vi "init.vi"(0 "VISA Refnum in":refnum<visa-resource-name>) -> (4 "VISA out":refnum<visa-resource-name>, 6 "client handle out":T2, 8 "Internet OK":bool, 10 "Cluster of queues":T1, 15 "VISA error out":errorcluster)   [LabVIEW 2016]
uses:
  <vilib>/httpClient/ClientHandle.ctl
  <vilib>/Utility/error.llb/DialogType.ctl
  <vilib>/Instr/_visa.llb/VISA Configure Serial Port (Instr).vi
  <vilib>/httpClient/LabVIEWHTTPClient.lvlib
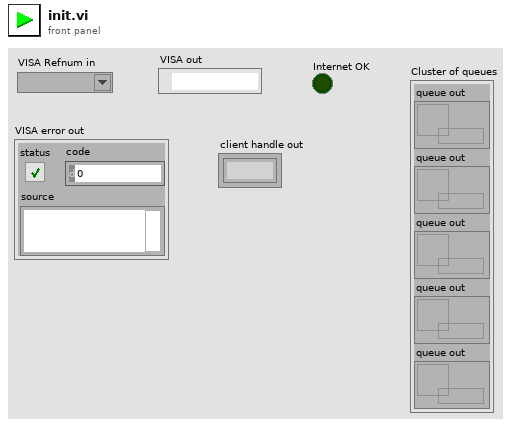
[diagram p1: front panel]
types:
  T1 = cluster{"queue out":refnum<queue>, "queue out":refnum<queue>, "queue out":refnum<queue>, "queue out":refnum<queue>, "queue out":refnum<queue>}
  T2 = typedef "LabVIEWHTTPClient.lvlib/ClientHandle.ctl" = refnum<k1>
  T3 = typedef "DialogType.ctl" = u16
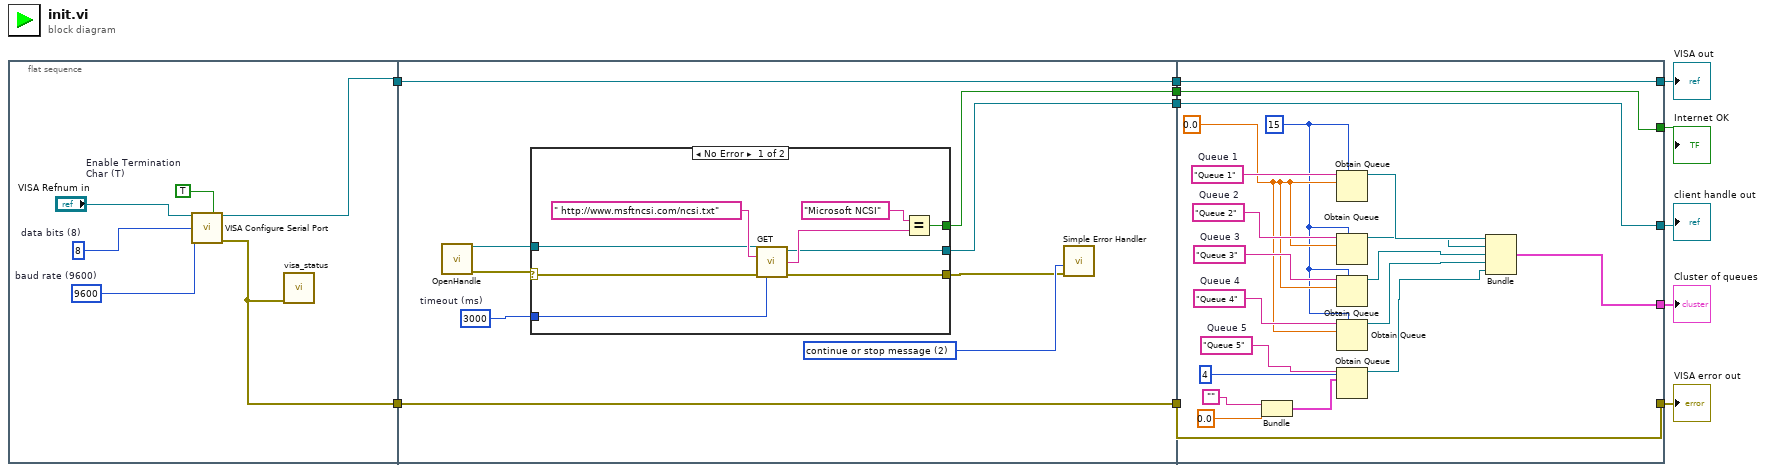
[diagram p0: block diagram]
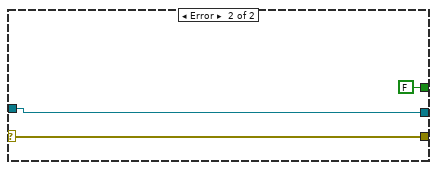
[diagram p2: hidden frame]
diagram:
  n1 = flat-sequence {
    tunnel: [w13] -> w11
    tunnel: [w12] -> w7
    tunnel: w11 -> [w21]
    tunnel: [w21] -> w10
    tunnel: [w20] -> w8
    tunnel: w7 -> [w20]
    tunnel: [w19] -> w5
    tunnel: [w18] -> w3
    tunnel: [w55] -> w9
    tunnel: w10 -> [w55]
    tunnel: [w54] -> w6
    tunnel: w8 -> [w54]
    tunnel: [w53] -> w4
    tunnel: w5 -> [w53]
    tunnel: [w52] -> w2
    tunnel: w3 -> [w52]
    tunnel: [w40] -> w1
    frame #0 {
      w14 = u16 8  # data bits (8)
      w15 = TRUE  # Enable Termination Char (T)
      w16 = u32 9600  # baud rate (9600)
      n2 = call-poly "VISA Configure Serial Port"("VISA resource name"="VISA Refnum in", "Enable Termination\nChar (T)"=w15, "baud rate (9600)"=w16, "data bits (8)"=w14) -> ("VISA resource name out"=w13:refnum<visa-resource-name>, "error out"=w12:errorcluster)  [unwired: 10 in]
      n3 = call "visa_status.vi"("error in (no error)"=w12) -> ()  [unwired: 11 in]
    }
    frame #1 {
      w23 = T3 2 items=["no dialog", "OK message", "continue or stop message", "OK message + warnings", "continue/stop + warnings"] ("type of dialog (OK msg:1)")
      w26 = 3000  # timeout (ms)
      n4 = call <vilib>:"OpenHandle.vi"() -> ("client handle out"=w24:T2, "error out"=w25:errorcluster)  [unwired: 14 in]
      n5 = case shown="No Error" w25 {
        selector: w25 -> [w30 w37]
        tunnel: [w32 FALSE] -> w19
        tunnel: [w31 w37] -> w22
        tunnel: w26 -> [w29 _]
        tunnel: w24 -> [w28 w36]
        tunnel: [w27 w36] -> w18
        frame No Error {
          n6 = call <vilib>:"GET.vi"("client handle"=w28, "url"=" http://www.msftncsi.com/ncsi.txt" ("address"), "error in (no error)"=w30, "timeout (10000)"=w29) -> ("client handle out"=w27:T2, "body"=w33:string, "error out"=w31:errorcluster)  [unwired: 8 in, 1 out]
          n7 = Equal?(x="Microsoft NCSI", y=w33) -> (x = y?=w32:bool)
        }
        frame Error {
        }
      }
      n8 = call <vilib>:"Simple Error Handler.vi"("type of dialog (OK msg:1)"=w23, "error in (no error)"=w22) -> ()  [unwired: 3 in, 5 out]
    }
    frame #2 {
      w50 = "Queue 5"  # Queue 5
      w49 = "Queue 4"  # Queue 4
      w51 = "Queue 3"  # Queue 3
      w48 = 0.0
      w44 = 15 ("max queue size (-1, unlimited)")
      w59 = "Queue 2"  # Queue 2
      w58 = "Queue 1"  # Queue 1
      n9 = Bundle("", 0.0) -> (w43:cluster{string, dbl})  [unwired: 1 in]
      n10 = Obtain Queue(max queue size (-1, unlimited)=w44, name (unnamed)=w58, element data type=w48) -> (queue out=w57:refnum<queue>)  [unwired: 2 in, 2 out]
      n11 = Obtain Queue(max queue size (-1, unlimited)=w44, name (unnamed)=w59, element data type=w48) -> (queue out=w56:refnum<queue>)  [unwired: 2 in, 2 out]
      n12 = Obtain Queue(max queue size (-1, unlimited)=w44, name (unnamed)=w51, element data type=w48) -> (queue out=w46:refnum<queue>)  [unwired: 2 in, 2 out]
      n13 = Obtain Queue(max queue size (-1, unlimited)=w44, name (unnamed)=w49, element data type=w48) -> (queue out=w45:refnum<queue>)  [unwired: 2 in, 2 out]
      n14 = Obtain Queue(max queue size (-1, unlimited)=4, name (unnamed)=w50, element data type=w43) -> (queue out=w41:refnum<queue>)  [unwired: 2 in, 2 out]
      n15 = Bundle("queue out"=w57, "queue out"=w56, "queue out"=w46, "queue out"=w45, "queue out"=w41) -> (w40:T1)  [unwired: 1 in]
    }
  }
  "VISA out" <- w9
  "VISA error out" <- w6
  "Internet OK" <- w4
  "client handle out" <- w2
  "Cluster of queues" <- w1
